vi "EF_CalcTimeTraceResolution.vi"(10 "BitShift":i32, 11 "Rate [Hz]":i32) -> (3 "DeltaT [ms]":dbl)   [LabVIEW 2017]
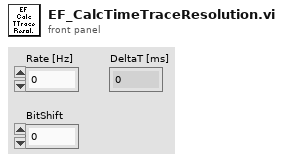
[diagram p1: front panel]
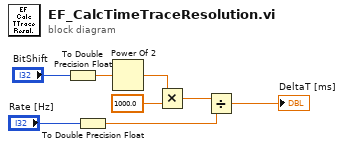
[diagram p0: block diagram]
diagram:
  n1 = To Double Precision Float(number="BitShift") -> (double precision float=w2:dbl)
  n2 = To Double Precision Float(number="Rate [Hz]") -> (double precision float=w4:dbl)
  n3 = Power Of 2(x=w2) -> (2^x=w5:dbl)
  n4 = Multiply(x=w5, y=1000.0) -> (x*y=w6:dbl)
  n5 = Divide(x=w6, y=w4) -> (x/y=→"DeltaT [ms]":dbl)
